vi "RIO_DoMath.vi"(2 "Stack in":string[](array[string]), 3 "Last Operation":string, 4 "URAPI Script":T1={"Script"="", "Whiles"=[], "Ifs"=[], "Supress Err"=TRUE, "Errors"=""}) -> (0 "Stack out":string[](array[string]), 1 "URAPI Script Out":T1={"Script"="", "Whiles"=[], "Ifs"=[], "Supress Err"=TRUE, "Errors"=""})   [LabVIEW 2012]
uses:
  <userlib>/BotSpeak/VIs/Direct/URAPI_Control.ctl
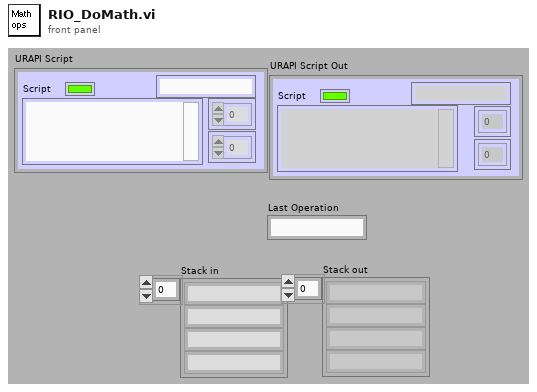
[diagram p1: front panel]
types:
  T1 = typedef "URAPI_Control.ctl" = cluster{"Script":string, "Whiles":u8[], "Ifs":u8[], "Supress Err":bool, "Errors":string}
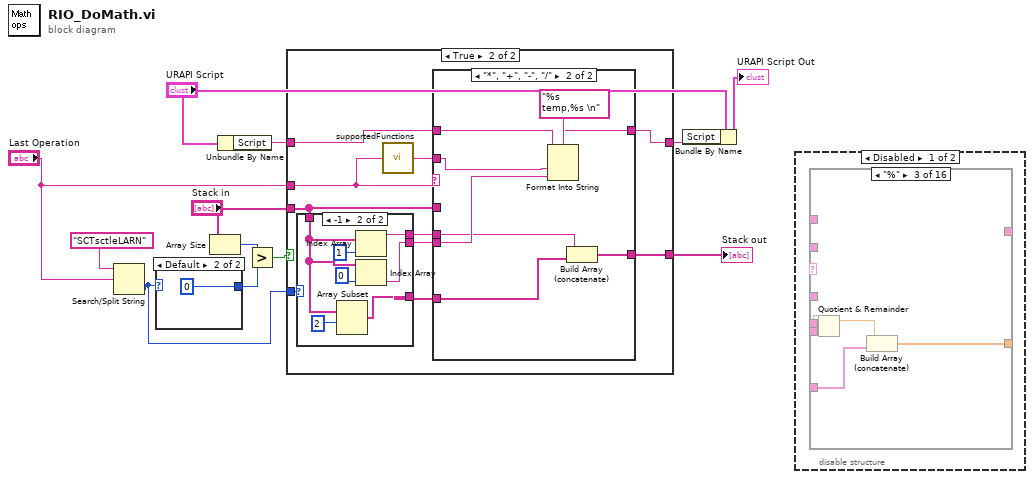
[diagram p0: block diagram]
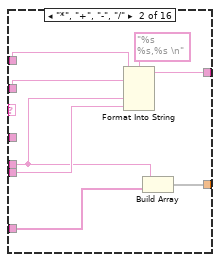
[diagram p3: hidden frame]
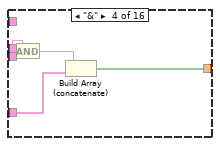
[diagram p4: hidden frame]
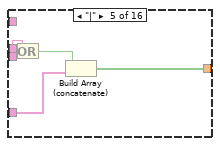
[diagram p5: hidden frame]
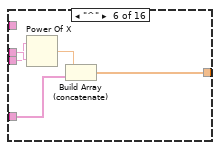
[diagram p6: hidden frame]
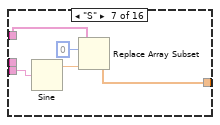
[diagram p7: hidden frame]
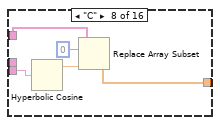
[diagram p8: hidden frame]
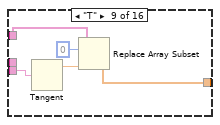
[diagram p9: hidden frame]
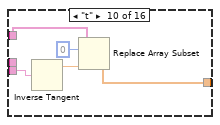
[diagram p10: hidden frame]
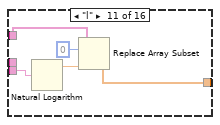
[diagram p11: hidden frame]
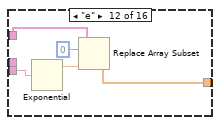
[diagram p12: hidden frame]
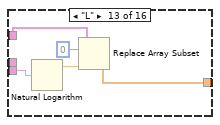
[diagram p13: hidden frame]
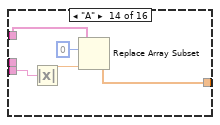
[diagram p14: hidden frame]
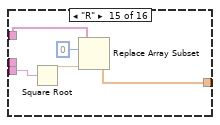
[diagram p15: hidden frame]
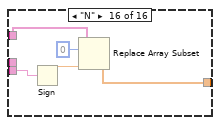
[diagram p16: hidden frame]
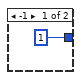
[diagram p18: hidden frame]
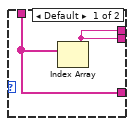
[diagram p20: hidden frame]
diagram:
  n1 = Search/Split String(string="SCTsctleLARN" ("String"), search string/char (-)="Last Operation") -> (offset of match=w6:i32)  [unwired: 1 in, 2 out]
  n2 = case shown="Default" w6 {
    tunnel: [1 ("y") 0 ("y")] -> w9
    frame -1 {
    }
    frame Default {
    }
  }
  n3 = Array Size(array="Stack in") -> (size(s)=w10:i32)
  n4 = Unbundle By Name("URAPI Script") -> ("Script"=w2:string)
  n5 = Greater?(x=w10, y=w9) -> (0:w8:bool)
  n6 = case shown="True" w8 {
    tunnel: "Last Operation" -> [_ w19]
    tunnel: [w16 w25] -> w12
    tunnel: "Stack in" -> [w16 w24]
    tunnel: w6 -> [_ w23]
    tunnel: w2 -> [w15 w20]
    tunnel: [w15 w17] -> w1
    frame False {
    }
    frame True {
      n7 = case shown="-1" w23 {
        tunnel: [w28 w34] -> w26
        tunnel: w24 -> [w28 w31]
        tunnel: [w27 w30] -> w22
        tunnel: [w27 w29] -> w21
        frame Default {
          n8 = Index Array(array=w28) -> (element=w27:string)  [unwired: 1 in]
        }
        frame -1 {
          n9 = Array Subset(array=w31, index=2 ("length")) -> (w34:string[])  [unwired: 1 in]
          n10 = Index Array(array=w31, index=1) -> (element=w30:string)
          n11 = Index Array(array=w31, index=0) -> (element=w29:string)
        }
      }
      n12 = call <userlib>:"supportedFunctions.vi"("String"=w19) -> ("regular expression"=w18:string)
      n13 = case shown="\"*\", \"+\", \"-\", \"/\"" w19 {
        tunnel: w22 -> [_ w39]
        tunnel: w21 -> [_ w41]
        tunnel: w26 -> [_ w45]
        tunnel: [w37 w44] -> w25
        tunnel: w24 -> [w37 _]
        tunnel: w20 -> [w36 w43]
        tunnel: w18 -> [_ w38]
        tunnel: [w36 w40] -> w17
        frame Default {
        }
        frame "*", "+", "-", "/" {
          n14 = Format Into String(format string="%s temp,%s \n", initial string=w43, w38, w41) -> (resulting string=w40:string)  [unwired: 1 in, 1 out]
          n15 = Build Array (concatenate)(w39, w45) -> (w44:string[])
        }
      }
    }
  }
  "Stack out" <- w12
  n16 = Bundle By Name(cluster="URAPI Script", "Script"=w1) -> (→"URAPI Script Out":T1)
  n17 = disable-structure shown="Disabled" {
    frame Disabled {
      n18 = case shown="\"%\"" {
        selector: _ -> [_ _ _ _ _ _ _ _ _ _ _ _ _ _ _ _]
        tunnel: _ -> [_ w47 w59 w64 w69 w72 _ _ _ _ _ _ _ _ _ _]
        tunnel: _ -> [_ w49 w58 w63 w68 w71 w79 w84 w89 w94 w99 w104 w109 w114 w119 w124]
        tunnel: _ -> [_ w54 w57 w62 w67 w74 _ _ _ _ _ _ _ _ _ _]
        tunnel: [w46 w53 w56 w61 w66 w73 w76 w81 w86 w91 w96 w101 w106 w111 w116 w121] -> _
        tunnel: _ -> [w46 _ _ _ _ _ w78 w83 w88 w93 w98 w103 w108 w113 w118 w123]
        tunnel: _ -> [_ w52 _ _ _ _ _ _ _ _ _ _ _ _ _ _]
        tunnel: _ -> [_ w50 _ _ _ _ _ _ _ _ _ _ _ _ _ _]
        tunnel: [_ w48 _ _ _ _ _ _ _ _ _ _ _ _ _ _] -> _
        frame Default {
        }
        frame "*", "+", "-", "/" {
          n19 = Format Into String(format string="%s %s,%s \n", initial string=w52, w50, w47, w49) -> (resulting string=w48:string)  [unwired: 1 in, 1 out]
          n20 = Build Array(w47, w54) -> (w53:void[])
        }
        frame "%" {
          n21 = Quotient & Remainder(x=w59, y=w58) -> (x-y*floor(x/y)=w55:dbl)  [unwired: 1 out]
          n22 = Build Array (concatenate)(w55, w57) -> (w56:dbl[])
        }
        frame "&" {
          n23 = And(x=w64, y=w63) -> (x .and. y?=w60:bool)
          n24 = Build Array (concatenate)(w60, w62) -> (w61:bool[])
        }
        frame "|" {
          n25 = Or(x=w69, y=w68) -> (x .or. y?=w65:bool)
          n26 = Build Array (concatenate)(w65, w67) -> (w66:bool[])
        }
        frame "^" {
          n27 = Power Of X(1:w72, 2:w71) -> (0:w70:dbl)
          n28 = Build Array (concatenate)(w70, w74) -> (w73:dbl[])
        }
        frame "S" {
          n29 = Sine(x=w79) -> (sin(x)=w77:dbl)
          n30 = Replace Array Subset(array=w78, new element=w77, index=0) -> (w76:dbl[])
        }
        frame "C" {
          n31 = Hyperbolic Cosine(1:w84) -> (0:w82:dbl)
          n32 = Replace Array Subset(array=w83, new element=w82, index=0) -> (w81:dbl[])
        }
        frame "T" {
          n33 = Tangent(1:w89) -> (0:w87:dbl)
          n34 = Replace Array Subset(array=w88, new element=w87, index=0) -> (w86:dbl[])
        }
        frame "t" {
          n35 = Inverse Tangent(1:w94) -> (0:w92:dbl)
          n36 = Replace Array Subset(array=w93, new element=w92, index=0) -> (w91:dbl[])
        }
        frame "l" {
          n37 = Natural Logarithm(1:w99) -> (0:w97:dbl)
          n38 = Replace Array Subset(array=w98, new element=w97, index=0) -> (w96:dbl[])
        }
        frame "e" {
          n39 = Exponential(1:w104) -> (0:w102:dbl)
          n40 = Replace Array Subset(array=w103, new element=w102, index=0) -> (w101:dbl[])
        }
        frame "L" {
          n41 = Natural Logarithm(1:w109) -> (0:w107:dbl)
          n42 = Replace Array Subset(array=w108, new element=w107, index=0) -> (w106:dbl[])
        }
        frame "A" {
          n43 = Absolute Value(x=w114) -> (abs(x)=w112:dbl)
          n44 = Replace Array Subset(array=w113, new element=w112, index=0) -> (w111:dbl[])
        }
        frame "R" {
          n45 = Square Root(x=w119) -> (sqrt(x)=w117:dbl)
          n46 = Replace Array Subset(array=w118, new element=w117, index=0) -> (w116:dbl[])
        }
        frame "N" {
          n47 = Sign(1:w124) -> (0:w122:dbl)
          n48 = Replace Array Subset(array=w123, new element=w122, index=0) -> (w121:dbl[])
        }
      }
    }
    frame Enabled {
    }
  }
